vi "Lifting Encoder Calculations.vi"(7 "Position":enum16{"0", "1", "2", "3", "4"}(ring), 10 "distance traveled":dbl) -> (1 "Current position":i32, 2 "Direction":enum16{"stop", "up", "down"}(ring)=enum."up")   [LabVIEW 2014]
panel:
  in  "Limit switch top":bool
  in  "Limit switch bottom":bool
  in  "Distance 3(2)":dbl
  in  "Distance 2(2)":dbl
  in  "Distance 1(2)":dbl
  in  "Distance 3":dbl
  in  "Distance 2":dbl
  in  "Distance 1":dbl
  # "Ranges"
  # "smaller"
  # "Larger"
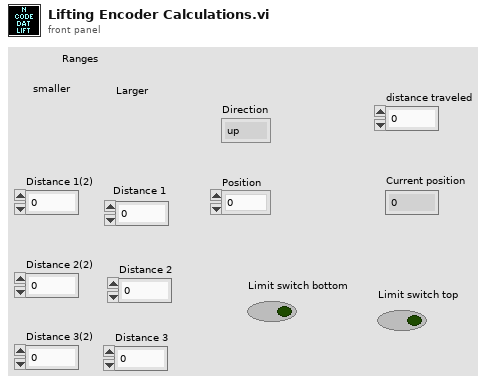
[diagram p1: front panel]
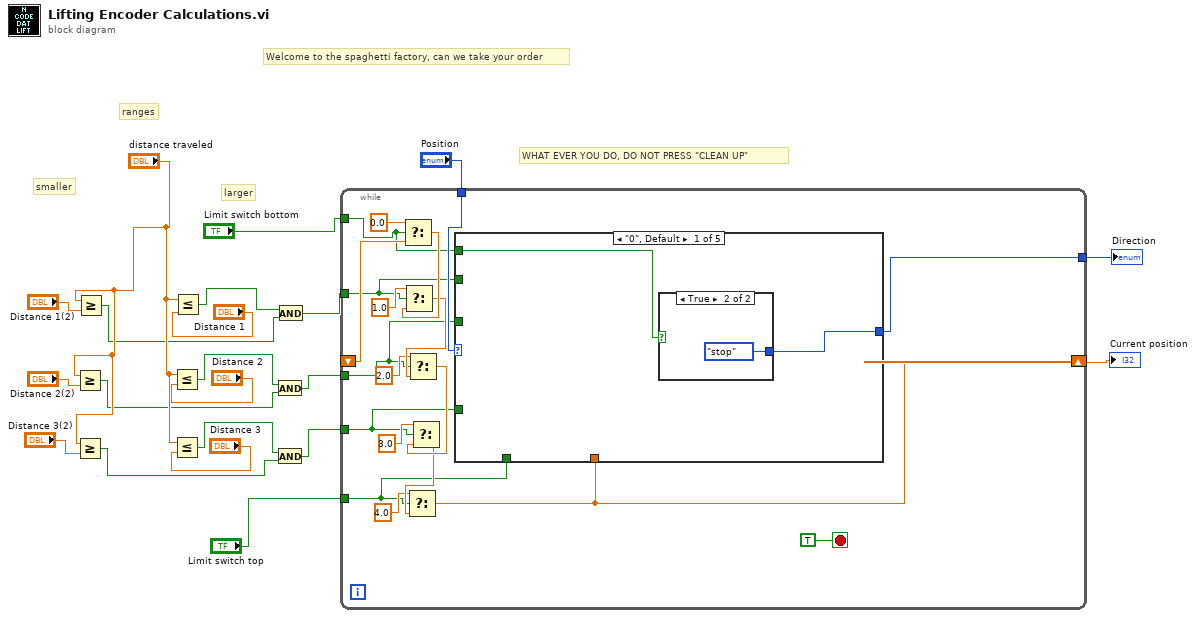
[diagram p0: block diagram]
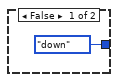
[diagram p2: hidden frame]
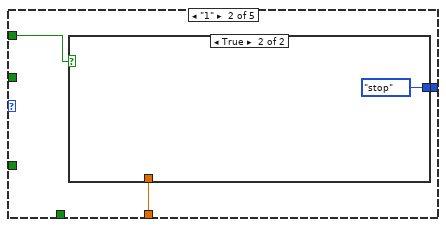
[diagram p3: hidden frame]
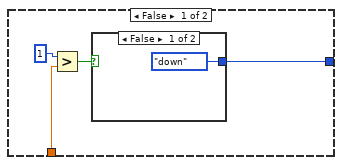
[diagram p4: hidden frame]
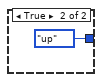
[diagram p5: hidden frame]
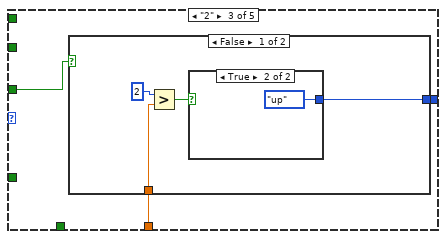
[diagram p6: hidden frame]
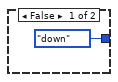
[diagram p7: hidden frame]
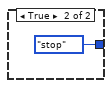
[diagram p8: hidden frame]
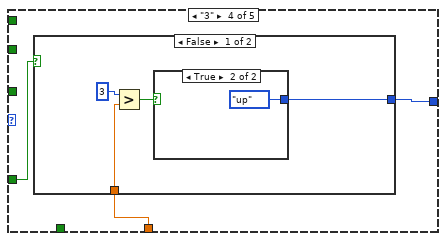
[diagram p9: hidden frame]
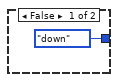
[diagram p10: hidden frame]
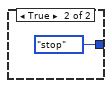
[diagram p11: hidden frame]
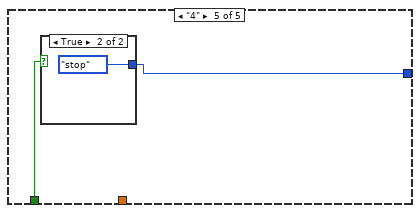
[diagram p12: hidden frame]
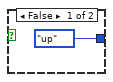
[diagram p13: hidden frame]
diagram:
  # "Welcome to the spaghetti factory, can we take your order"
  # "WHAT EVER YOU DO, DO NOT PRESS \"CLEAN UP\""
  # "larger"
  # "smaller"
  # "ranges"
  n1 = Greater Or Equal?(x="distance traveled", y="Distance 2(2)") -> (x >= y?=w8:bool)
  n2 = Greater Or Equal?(x="distance traveled", y="Distance 3(2)") -> (x >= y?=w7:bool)
  n3 = Greater Or Equal?(x="distance traveled", y="Distance 1(2)") -> (x >= y?=w9:bool)
  n4 = Less Or Equal?(x="distance traveled", y="Distance 2") -> (x <= y?=w11:bool)
  n5 = Less Or Equal?(x="distance traveled", y="Distance 3") -> (x <= y?=w12:bool)
  n6 = Less Or Equal?(x="distance traveled", y="Distance 1") -> (x <= y?=w10:bool)
  n7 = And(x=w11, y=w8) -> (x .and. y?=w5:bool)
  n8 = And(x=w12, y=w7) -> (x .and. y?=w4:bool)
  n9 = And(x=w10, y=w9) -> (x .and. y?=w6:bool)
  n10 = while {
    shift-right: [w24] -> w3
    shift-left: _ -> [w29]
    tunnel: [w39] -> w21
    tunnel: "Position" -> [w38]
    tunnel: w6 -> [w27]
    tunnel: w5 -> [w26]
    tunnel: w4 -> [w25]
    tunnel: "Limit switch top" -> [w22]
    tunnel: "Limit switch bottom" -> [w23]
    stop <- TRUE stop-if-true
    n11 = Select(t=0.0, s=w23, f=w29) -> (s? t:f=w37:dbl)
    n12 = Select(t=1.0 ("f"), s=w27, f=w37) -> (s? t:f=w36:dbl)
    n13 = Select(t=2.0 ("f"), s=w26, f=w36) -> (s? t:f=w35:dbl)
    n14 = Select(t=3.0 ("f"), s=w25, f=w35) -> (s? t:f=w34:dbl)
    n15 = Select(t=4.0 ("f"), s=w22, f=w34) -> (s? t:f=w24:dbl)
    n16 = case shown="\"0\", Default" w38 {
      tunnel: [w42 w47 w57 w67 w76] -> w39
      tunnel: w24 -> [_ w46 w56 w66 _]
      tunnel: w23 -> [w41 _ _ _ _]
      tunnel: w27 -> [_ w45 _ _ _]
      tunnel: w26 -> [_ _ w55 _ _]
      tunnel: w25 -> [_ _ _ w65 _]
      tunnel: w22 -> [_ _ _ _ w75]
      frame "0", Default {
        n17 = case shown="True" w41 {
          tunnel: [enum16{"stop", "up", "down"}."down" ("Direction") enum16{"stop", "up", "down"}."stop" ("Direction")] -> w42
          frame False {
          }
          frame True {
          }
        }
      }
      frame "1" {
        n18 = case shown="True" w45 {
          tunnel: [w51 enum16{"stop", "up", "down"}."stop" ("Direction")] -> w47
          tunnel: w46 -> [w48 _]
          frame False {
            n19 = Greater?(x=1, y=w48) -> (0:w49:bool)
            n20 = case shown="False" w49 {
              tunnel: [enum16{"stop", "up", "down"}."down" ("Direction") enum16{"stop", "up", "down"}."up" ("Direction")] -> w51
              frame False {
              }
              frame True {
              }
            }
          }
          frame True {
          }
        }
      }
      frame "2" {
        n21 = case shown="False" w55 {
          tunnel: [w61 enum16{"stop", "up", "down"}."stop" ("Direction")] -> w57
          tunnel: w56 -> [w58 _]
          frame False {
            n22 = Greater?(x=2, y=w58) -> (0:w60:bool)
            n23 = case shown="True" w60 {
              tunnel: [enum16{"stop", "up", "down"}."down" ("Direction") enum16{"stop", "up", "down"}."up" ("Direction")] -> w61
              frame False {
              }
              frame True {
              }
            }
          }
          frame True {
          }
        }
      }
      frame "3" {
        n24 = case shown="False" w65 {
          tunnel: [w71 enum16{"stop", "up", "down"}."stop" ("Direction")] -> w67
          tunnel: w66 -> [w68 _]
          frame False {
            n25 = Greater?(x=3, y=w68) -> (0:w70:bool)
            n26 = case shown="True" w70 {
              tunnel: [enum16{"stop", "up", "down"}."down" ("Direction") enum16{"stop", "up", "down"}."up" ("Direction")] -> w71
              frame False {
              }
              frame True {
              }
            }
          }
          frame True {
          }
        }
      }
      frame "4" {
        n27 = case shown="True" w75 {
          tunnel: [enum16{"stop", "up", "down"}."up" ("Direction") enum16{"stop", "up", "down"}."stop" ("Direction")] -> w76
          frame False {
          }
          frame True {
          }
        }
      }
    }
  }
  "Direction" <- w21
  "Current position" <- w3
